vi "constructor.vi"(8 "error in (no error)":errorcluster, 9 "deviceDataBase":refnum<class "deviceDataBase.lvclass">, 10 "Path":path, 11 "compiledTime":timestamp) -> (0 "error out":errorcluster, 1 "error":bool, 2 "DeviceArray":refnum<class "DeviceArray.lvclass">, 3 "ScriptListCompiler out":refnum<class "ScriptListCompiler.lvclass">)   [LabVIEW 2011, in "Compiler.lvlib" / "ScriptListCompiler.lvclass"]
uses:
  ScriptListCompiler.lvclass
  DatabaseHelpers/DbConnection/DeviceDataBase/deviceDataBase.lvclass
  DatabaseHelpers/Database Objects/DeviceArray/DeviceArray.lvclass
  Scripting/DataPointScript/DataPointScript.lvclass
  ScriptListCompiler.lvclass/ScriptListCompiler.ctl
  Scripting/ScriptingEvent/ScriptEventList/ScriptEventList.lvclass
  Compiler.lvlib
panel:
  out "openTime":dbl
  out "load Time":dbl
  out "compileTime":dbl
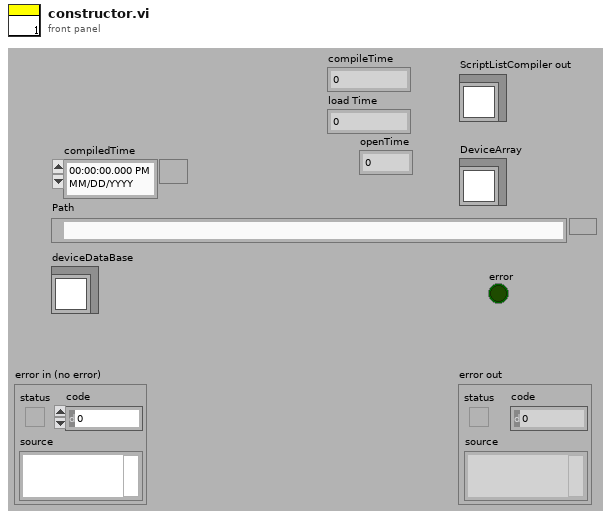
[diagram p1: front panel]
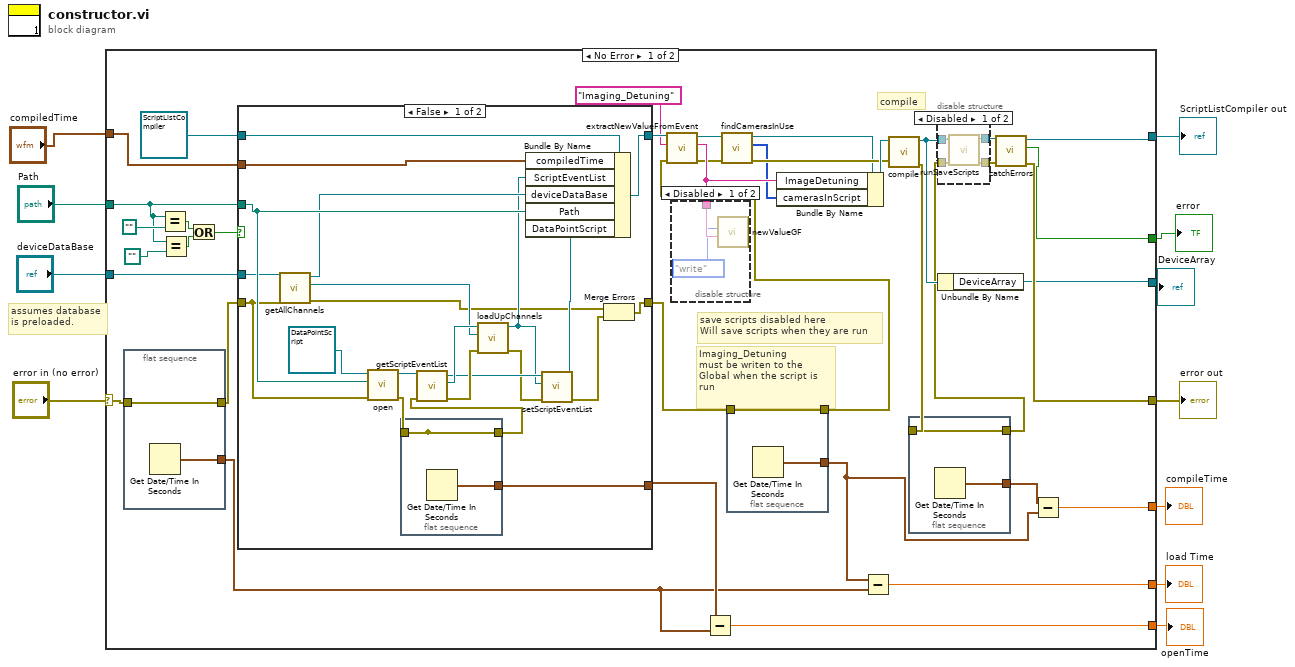
[diagram p0: block diagram]
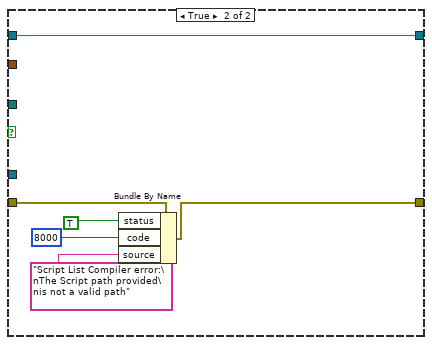
[diagram p4: hidden frame]
diagram:
  # "assumes database\nis preloaded."
  n1 = case shown="No Error" "error in (no error)" {
    selector: "error in (no error)" -> [w23 w94]
    tunnel: [w40 w94] -> w10
    tunnel: [w41 _] -> w7
    tunnel: "Path" -> [w42 _]
    tunnel: "deviceDataBase" -> [w45 _]
    tunnel: [w39 _] -> w6
    tunnel: "compiledTime" -> [w38 _]
    tunnel: [w37 _] -> w5
    tunnel: [w16 _] -> w3
    tunnel: [w15 _] -> w2
    tunnel: [w12 _] -> w1
    frame No Error {
      # "Imaging_Detuning\nmust be writen to the\nGlobal when the script is run"
      # "save scripts disabled here\nWill save scripts when they are run"
      # "compile"
      n2 = flat-sequence {
        tunnel: [w55] -> w24
        tunnel: w23 -> [w55]
        tunnel: [w54] -> w13
        frame #0 {
          n3 = Get Date/Time In Seconds() -> (seconds since 1Jan1904=w54:timestamp)
        }
      }
      n4 = Equal?(x=w42, y=path "") -> (x = y?=w48:bool)
      n5 = Equal?(x=w42, y=path "") -> (x = y?=w47:bool)
      n6 = Or(x=w48, y=w47) -> (x .or. y?=w44:bool)
      n7 = case shown="False" w44 {
        tunnel: w45 -> [w78 _]
        tunnel: refnum<class "ScriptListCompiler.lvclass"> refnum ("SettingsProcessors.lvlib:ScriptListCompiler.lvclass") -> [w85 w88]
        tunnel: [w84 w88] -> w36
        tunnel: w42 -> [w79 _]
        tunnel: w24 -> [w76 w93]
        tunnel: [w70 w92] -> w22
        tunnel: w38 -> [w67 _]
        tunnel: [w64 _] -> w14
        frame False {
          n8 = call "getAllChannels.vi"("error in (no error)"=w76, "deviceDataBase in"=w78) -> ("error out"=w69:errorcluster, "ChannelArray.lvclass"=w75:refnum<class "ChannelArray.lvclass">, "deviceDataBase out"=w77:refnum<class "deviceDataBase.lvclass">)  [unwired: 7 in]
          n9 = call "open.vi"("error in (no error)"=w76, "Path"=w79, "DataPointScript in"=refnum<class "DataPointScript.lvclass"> refnum ("Tools.lvlib:Scripting.lvlib:DataPointScript.lvclass")) -> ("error out"=w66:errorcluster, "DataPointScript out"=w82:refnum<class "DataPointScript.lvclass">)  [unwired: 7 in]
          n10 = flat-sequence {
            tunnel: [w86] -> w65
            tunnel: [w86] -> _
            tunnel: [w87] -> w64
            tunnel: w66 -> [w86]
            frame #0 {
              n11 = Get Date/Time In Seconds() -> (seconds since 1Jan1904=w87:timestamp)
            }
          }
          n12 = call "getScriptEventList.vi"("error in (no error)"=w65, "DataPointScript.lvclass in"=w82) -> ("error out"=w80:errorcluster, "ScriptEventList"=w81:refnum<class "ScriptEventList.lvclass">, "DataPointScript.lvclass out"=w74:refnum<class "DataPointScript.lvclass">)  [unwired: 7 in]
          n13 = call "loadUpChannels.vi"("error in (no error)"=w80, "ChannelArray"=w75, "ScriptEventList in"=w81) -> ("error out"=w73:errorcluster, "ScriptEventList out"=w72:refnum<class "ScriptEventList.lvclass">)  [unwired: 7 in]
          n14 = call "setScriptEventList.vi"("error in (no error)"=w73, "TScriptEventList"=w72, "DataPointScript.lvclass in"=w74) -> ("error out"=w68:errorcluster, "DataPointScript.lvclass out"=w71:refnum<class "DataPointScript.lvclass">)  [unwired: 7 in]
          n15 = Bundle By Name(cluster=w85, "compiledTime"=w67, "ScriptEventList"=w72, "deviceDataBase"=w77, "Path"=w79, "DataPointScript"=w71) -> (w84:refnum<class "ScriptListCompiler.lvclass">)
          n16 = Merge Errors(w69, w68) -> (w70:errorcluster)
        }
        frame True {
          n17 = Bundle By Name(cluster=w93, "status"=TRUE, "code"=8000, "source"="Script List Compiler error:\nThe Script path provided\nis not a valid path") -> (w92:errorcluster)
        }
      }
      n18 = call "extractNewValueFromEvent.vi"("error in (no error)"=w21, "channelName"="Imaging_Detuning", "ScriptListCompiler in"=w36) -> ("error out"=w28:errorcluster, "newValue"=w30:string, "ScriptListCompiler out"=w29:refnum<class "ScriptListCompiler.lvclass">)  [unwired: 6 in]
      n19 = disable-structure shown="Disabled" {
        disable-tunnel: w30 -> [w57 _]
        frame Disabled {
          n20 = call "newValueGF.vi"("newValue"=w57, "control"=enum16{"read", "write"}."write") -> ()  [unwired: 9 in, 1 out]
        }
        frame Enabled {
        }
      }
      n21 = Subtract(x=w14, y=w13) -> (x-y=w12:dbl)
      n22 = call "findCamerasInUse.vi"("error in (no error)"=w28, "ScriptListCompiler in"=w29) -> ("error out"=w27:errorcluster, "camerasInScript"=w25:enum16{"Pixis", "ProEM", "PixelFly"}[], "ScriptListCompiler out"=w26:refnum<class "ScriptListCompiler.lvclass">)  [unwired: 7 in]
      n23 = flat-sequence {
        tunnel: [w53] -> w21
        tunnel: w22 -> [w53]
        tunnel: [w52] -> w17
        frame #0 {
          n24 = Get Date/Time In Seconds() -> (seconds since 1Jan1904=w52:timestamp)
        }
      }
      n25 = Bundle By Name(cluster=w26, "ImageDetuning"=w30, "camerasInScript"=w25) -> (w31:refnum<class "ScriptListCompiler.lvclass">)
      n26 = Subtract(x=w17, y=w13) -> (x-y=w15:dbl)
      n27 = call-dynamic "compile.vi"("error in (no error)"=w27, "ScriptListCompiler in"=w31) -> ("error out"=w20:errorcluster, "ScriptListCompiler out"=w33:refnum<class "ScriptListCompiler.lvclass">)  [unwired: 8 in]
      n28 = flat-sequence {
        tunnel: [w51] -> w19
        tunnel: w20 -> [w51]
        tunnel: [w50] -> w18
        frame #0 {
          n29 = Get Date/Time In Seconds() -> (seconds since 1Jan1904=w50:timestamp)
        }
      }
      n30 = disable-structure shown="Disabled" {
        disable-tunnel: [w61 w62] -> w34
        disable-tunnel: w19 -> [w60 w62]
        disable-tunnel: w33 -> [w59 w63]
        disable-tunnel: [w58 w63] -> w32
        frame Disabled {
          n31 = call "runSaveScripts.vi"("error in (no error)"=w60, "ScriptListCompiler in"=w59) -> ("error out"=w61:errorcluster, "ScriptListCompiler out"=w58:refnum<class "ScriptListCompiler.lvclass">)  [unwired: 8 in]
        }
        frame Enabled {
        }
      }
      n32 = Unbundle By Name(w33) -> ("DeviceArray"=w37:refnum<class "DeviceArray.lvclass">)
      n33 = call "catchErrors.vi"("error in (no error)"=w34, "ScriptListCompiler in"=w32) -> ("error out"=w40:errorcluster, "error"=w39:bool, "ScriptListCompiler out"=w41:refnum<class "ScriptListCompiler.lvclass">)  [unwired: 7 in]
      n34 = Subtract(x=w18, y=w17) -> (x-y=w16:dbl)
    }
    frame Error {
    }
  }
  "error out" <- w10
  "ScriptListCompiler out" <- w7
  "error" <- w6
  "DeviceArray" <- w5
  "compileTime" <- w3
  "load Time" <- w2
  "openTime" <- w1
